vi "hydraharp_set_binning.vi"(8 "error in (no error)":errorcluster, 10 "Binning":i32, 11 "hydraharp in":refnum<class "hydraharp.lvclass">) -> (0 "error out":errorcluster, 3 "hydraharp out":refnum<class "hydraharp.lvclass">)   [LabVIEW 2015, in "hydraharp.lvclass"]
uses:
  hydraharp.lvclass
  hydraharp.lvclass/hydraharp.ctl
  hhlib.dll
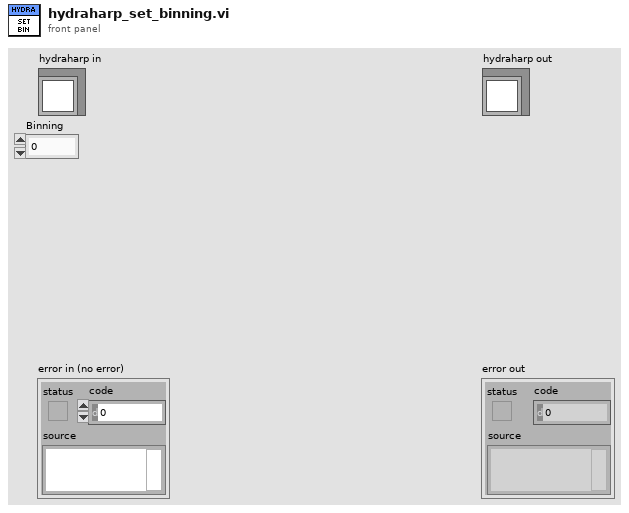
[diagram p1: front panel]
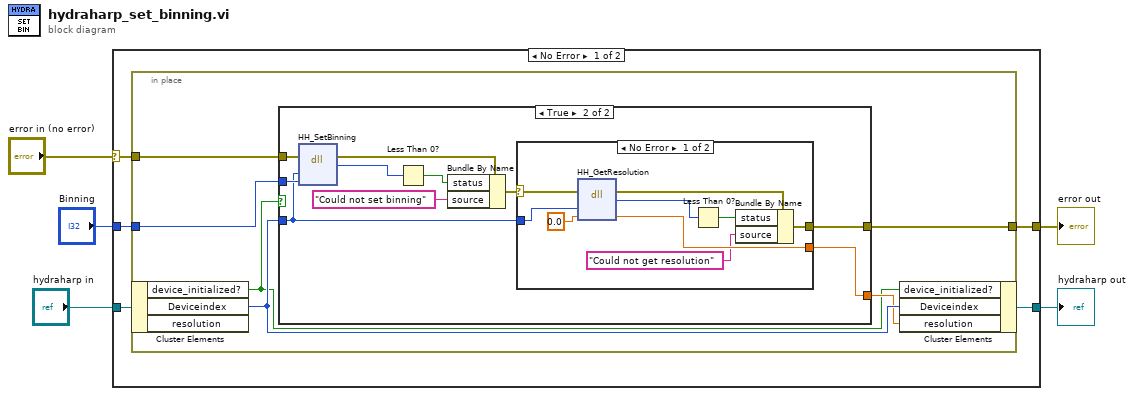
[diagram p0: block diagram]
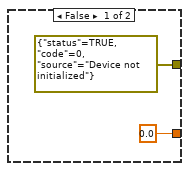
[diagram p2: hidden frame]
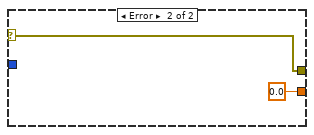
[diagram p3: hidden frame]
diagram:
  n1 = case shown="No Error" "error in (no error)" {
    selector: "error in (no error)" -> [w9 w41]
    tunnel: [w8 w41] -> w4
    tunnel: [w7 w40] -> w2
    tunnel: "hydraharp in" -> [w10 w40]
    tunnel: "Binning" -> [w6 _]
    frame No Error {
      n2 = in-place {
        in-place-border: w9 -> [w16]
        in-place-border: [w15] -> w8
        in-place-border: w6 -> [w14]
        n3 = in-place-cluster #1(w10) -> ("device_initialized?"=w11:bool, "Deviceindex"=w13:i32)  [unwired: 1 out]
        n4 = case shown="True" w11 {
          tunnel: w16 -> [_ w28]
          tunnel: [errorcluster {"status"=TRUE, "code"=0, "source"="Device not initialized"} ("error out") w26] -> w15
          tunnel: w14 -> [_ w25]
          tunnel: w13 -> [_ w24]
          tunnel: [0.0 ("resolution") w23] -> w12
          frame False {
          }
          frame True {
            n5 = dll-call lib="hhlib.dll" fn="HH_SetBinning"(error in=w28, "devidx"=w24, "Range"=w25) -> (error out=w22:errorcluster, w27:i32)  [unwired: 4 in, 1 out]
            n6 = Less Than 0?(x=w27) -> (x < 0?=w21:bool)
            n7 = Bundle By Name(cluster=w22, "status"=w21, "source"="Could not set binning") -> (w19:errorcluster)
            n8 = case shown="No Error" w19 {
              selector: w19 -> [w34 w38]
              tunnel: w24 -> [w37 _]
              tunnel: [w29 w38] -> w26
              tunnel: [w35 0.0 ("resolution")] -> w23
              frame No Error {
                n9 = dll-call lib="hhlib.dll" fn="HH_GetResolution"(error in=w34, "devidx"=w37, "resolution"=0.0) -> (error out=w32:errorcluster, w33:i32, "resolution"=w35:dbl)  [unwired: 3 in, 1 out]
                n10 = Less Than 0?(x=w33) -> (x < 0?=w31:bool)
                n11 = Bundle By Name(cluster=w32, "status"=w31, "source"="Could not get resolution") -> (w29:errorcluster)
              }
              frame Error {
              }
            }
          }
        }
        n12 = in-place-cluster #1("device_initialized?"=w11, "Deviceindex"=w13, "resolution"=w12) -> (w7:refnum<class "hydraharp.lvclass">)
      }
    }
    frame Error {
    }
  }
  "error out" <- w4
  "hydraharp out" <- w2
